vi "Create DS Alert.vi"(7 "group":string, 8 "error in (no error)":errorcluster, 10 "level":T1 items=["High", "Medium", "Low"], 11 "text":string) -> (0 "error out":errorcluster, 3 "handle out":i64)   [LabVIEW 2026, in "MrcLib.lvlib"]
doc: "Create a persistent alert that the DS and DBs can display for a summary of robot status."
uses:
  MrcLib.lvlib
  Alert Level.ctl
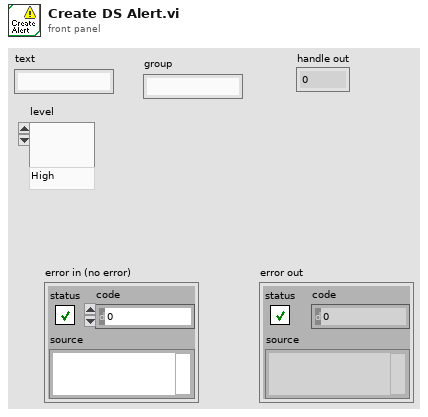
[diagram p1: front panel]
types:
  T1 = typedef "Alert Level.ctl" = u16
  T2 = typedef "MRC String.ctl" = cluster{"pointer":u64, "length":u64}
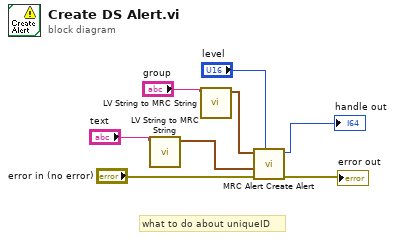
[diagram p0: block diagram]
diagram:
  # "what to do about uniqueID"
  n1 = call "LV String to MRC String.vi"("LV String"="text") -> ("MRC String"=w3:T2)  [unwired: 10 in]
  n2 = call "LV String to MRC String.vi"("LV String"="group") -> ("MRC String"=w5:T2)  [unwired: 10 in]
  n3 = call "MRC Alert Create Alert.vi"("level"="level", "error in (no error)"="error in (no error)", "text"=w3, "group"=w5) -> ("error out"=→"error out":errorcluster, "handle out"=→"handle out":i64)  [unwired: 6 in]
